vi "Create.vi"(10 "MessageQ":refnum<class "MessageQ.lvclass">) -> (3 "MessageQ Value out":refnum<class "MessageQ Value.lvclass">)   [LabVIEW 2020, in "Volatus.lvlib" / "MessageQ Value.lvclass"]
uses:
  MessageQ Value.lvclass
  MessageQ Value.lvclass/MessageQ Value.ctl
  MessageQ/MessageQ.lvclass
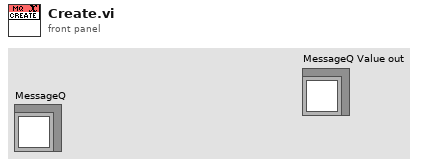
[diagram p1: front panel]
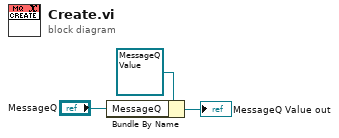
[diagram p0: block diagram]
diagram:
  n1 = Bundle By Name(cluster=refnum<class "MessageQ Value.lvclass"> refnum ("MessageQ Value in"), "MessageQ"="MessageQ") -> (→"MessageQ Value out":refnum<class "MessageQ Value.lvclass">)
